vi "Bitmap Glyph Data to Image.vi"(5 "Back":u32(colorbox)=16448250, 6 "Alpha":u8=255, 7 "Front":u32(colorbox), 8 "error in (no error)":errorcluster, 11 "Bitmap Glyph Rec":T2) -> (0 "error out":errorcluster, 3 "image data":T1)   [LabVIEW 2023, in "Freetype Drawer.lvlib"]
uses:
  Freetype Drawer.lvlib
  Bitmap Glyph.ctl
  Glyph Rec.ctl
  FT Bitmap.ctl
  <vilib>/picture/picture.llb/imagedata.ctl
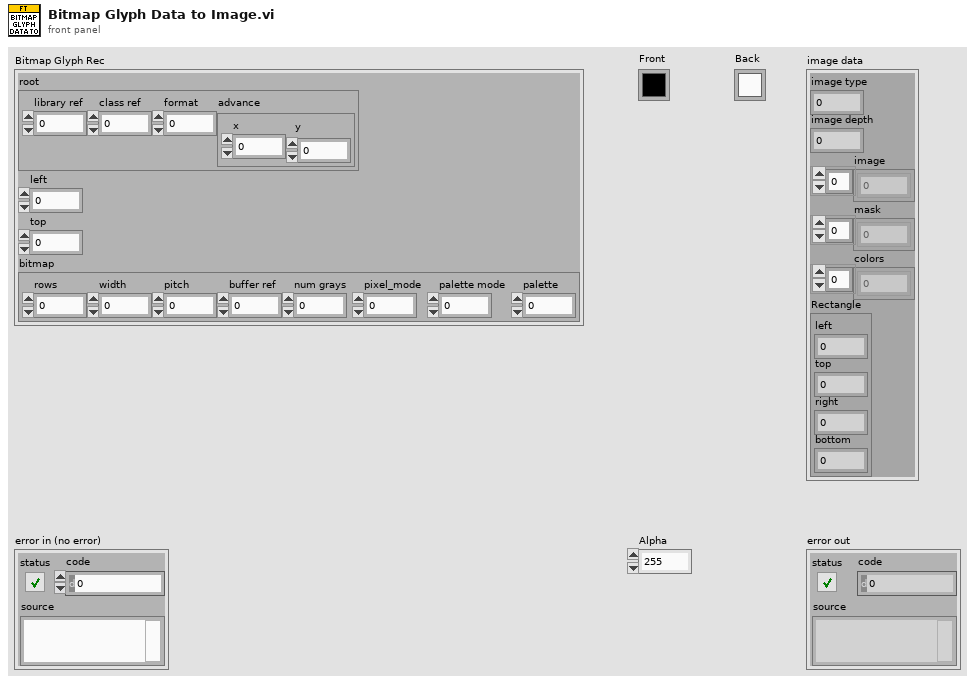
[diagram p1: front panel]
types:
  T1 = typedef "imagedata.ctl" = cluster{"image type":i32, "image depth":i32, "image":u8[], "mask":u8[], "colors":u32[], "Rectangle":cluster{"left":i16, "top":i16, "right":i16, "bottom":i16}}
  T2 = typedef "Freetype Drawer.lvlib/Bitmap Glyph.ctl" = cluster{"root":T3, "left":i32, "top":i32, "bitmap":T4}
  T3 = typedef "Freetype Drawer.lvlib/Glyph Rec.ctl" = cluster{"library ref":i64, "class ref":i64, "format":i32, "advance":cluster{"x":i32, "y":i32}}
  T4 = typedef "Freetype Drawer.lvlib/FT Bitmap.ctl" = cluster{"rows":u32, "width":u32, "pitch":i32, "buffer ref":i64, "num grays":i16, "pixel_mode":u8, "palette mode":u8, "palette":i64}
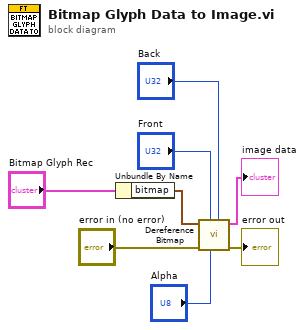
[diagram p0: block diagram]
diagram:
  n1 = Unbundle By Name("Bitmap Glyph Rec") -> ("bitmap"=w2:T4)
  n2 = call "Dereference Bitmap.vi"("Back"="Back", "Alpha"="Alpha", "Front"="Front", "error in (no error)"="error in (no error)", "bitmap"=w2) -> ("error out"=→"error out":errorcluster, "image data"=→"image data":T1)  [unwired: 5 in]
